vi "macro_DrumSeq_Continuous.vi"() -> ()   [LabVIEW 2019, in "Trajectory_Library.lvlib"]
uses:
  VI/BoolCmd_Recv_Internal.vi
  VI/DigSeqLogic_Edge_On.vi
  Util_GetTime.vi
  Timer_New.vi
  VI/BoolCmd_ObtainQueue.vi
  VI/Util_GetTime_U32.vi
  VI/Util_GetTime_U64.vi
  <vilib>/Utility/semaphor.llb/Obtain Semaphore Reference.vi
  Timer_Reset.vi
  VI/Timer_Restart.vi
  Timer_HasPeriodPassedOnce.vi
  Trajectory_Library.lvlib
panel:
  out "Some Speed demand":dbl
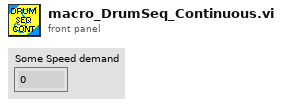
[diagram p1: front panel]
types:
  T1 = typedef "Trajectory_Library.lvlib/DrumSequence_Step_Enum.ctl" = enum16{"Do Nothing", "Step 1", "Step 2", "Step 3", "Step 4", "Step 5", "Step 6", "Step 7", "Step 8", "Step 9", "Step 10", "Step 11", "Step 12", "Step 13", "Step 14", "Step 15", "Step 16", "Step 17", "Step 18", "Step 19", "Step 20", "Step 21", "Step 22", "Step 23", "Step 24", "Step 25", "Step 26", "Step 27", "Step 28", "Step 29", "Step 30", "Step 31", "Step 32", "Cancel", "Initialize", "Error"}
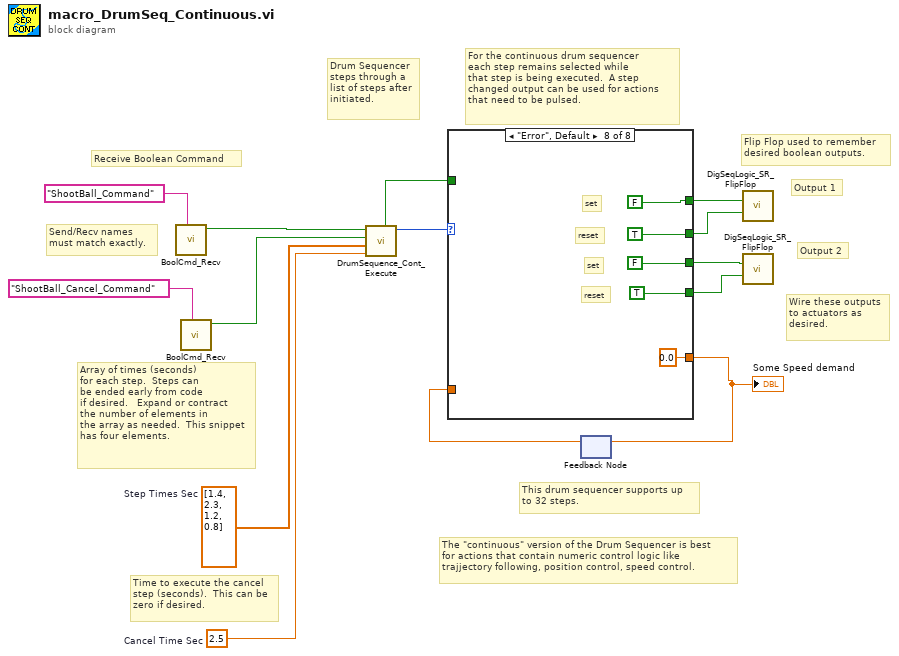
[diagram p0: block diagram]
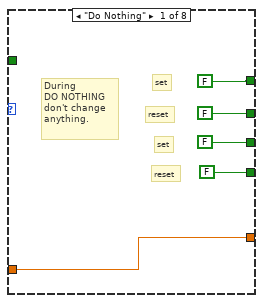
[diagram p2: hidden frame]
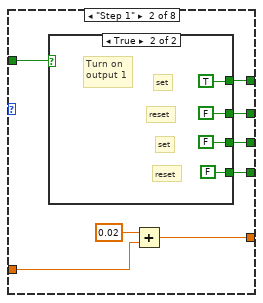
[diagram p3: hidden frame]
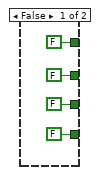
[diagram p4: hidden frame]
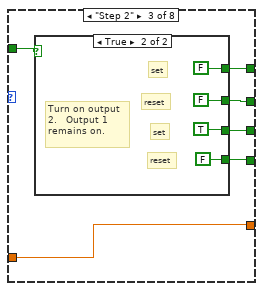
[diagram p5: hidden frame]
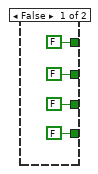
[diagram p6: hidden frame]
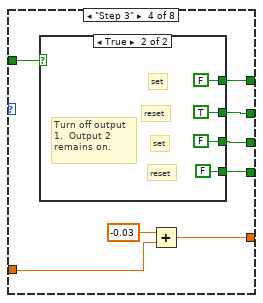
[diagram p7: hidden frame]
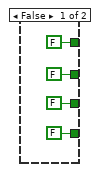
[diagram p8: hidden frame]
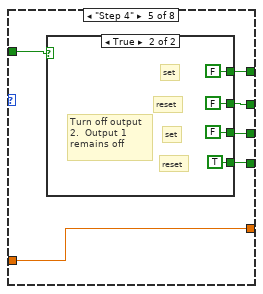
[diagram p9: hidden frame]
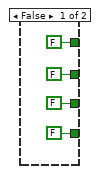
[diagram p10: hidden frame]
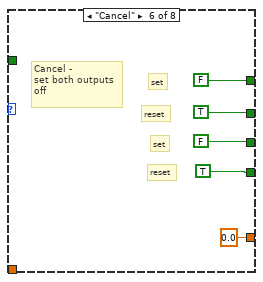
[diagram p11: hidden frame]
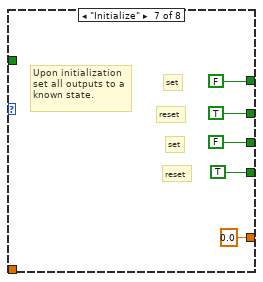
[diagram p12: hidden frame]
diagram:
  w9 = 2.5  # Cancel Time Sec
  w10 = dbl[] [1.4, 2.3, 1.2, 0.8]  # Step Times Sec
  # "This drum sequencer supports up\nto 32 steps."
  # "Wire these outputs\nto actuators as\ndesired."
  # "Output 2"
  # "Output 1"
  # "Flip Flop used to remember\ndesired boolean outputs."
  # "The \"continuous\" version of the Drum Sequencer is best\nfor actions that contain numeric control logic like \ntrajjectory following, position control, speed control."
  # "For the continuous drum sequencer\neach step remains selected while\nthat step is being executed.  A step\nchanged output can be used for actions\nthat need to be pulsed."
  # "Drum Sequencer\nsteps through a \nlist of steps after\ninitiated."
  # "Time to execute the cancel\nstep (seconds).  This can be\nzero if desired."
  # "Array of times (seconds)\nfor each step.  Steps can\nbe ended early from code\nif desired.   Expand or contract\nthe number of elements in\nthe array as needed.  This snippet\nhas four elements."
  # "Send/Recv names\nmust match exactly."
  # "Receive Boolean Command"
  n1 = call "BoolCmd_Recv.vi"("Command Name"="ShootBall_Command") -> ("New Request"=w13:bool)  [unwired: 9 in, 1 out]
  n2 = call "BoolCmd_Recv.vi"("Command Name"="ShootBall_Cancel_Command") -> ("New Request"=w11:bool)  [unwired: 9 in, 1 out]
  n3 = call "DrumSequence_Cont_Execute.vi"("Cancel Time Sec"=w9, "Step Times Sec"=w10, "Cancel"=w11, "Initiate"=w13) -> ("Step Number State"=w8:T1, "New Step"=w3:bool)  [unwired: 3 in, 3 out]
  n4 = feedback #1() -> (w1:dbl)  [unwired: 1 in]
  n5 = case shown="\"Error\", Default" w8 {
    tunnel: [FALSE w24 w38 w54 w68 FALSE FALSE FALSE] -> w7
    tunnel: [FALSE w25 w39 w55 w69 TRUE TRUE TRUE] -> w6
    tunnel: [FALSE w26 w40 w56 w70 FALSE FALSE FALSE] -> w5
    tunnel: [FALSE w27 w41 w57 w71 TRUE TRUE TRUE] -> w4
    tunnel: w3 -> [_ w23 w36 w50 w66 _ _ _]
    tunnel: [w15 w20 w37 w51 w67 0.0 0.0 0.0] -> w2
    tunnel: w1 -> [w15 w21 w37 w52 w67 _ _ _]
    frame "Do Nothing" {
      # "During \nDO NOTHING\ndon't change\nanything."
      # "reset"
      # "set"
      # "reset"
      # "set"
    }
    frame "Step 1" {
      n6 = case shown="True" w23 {
        tunnel: [FALSE FALSE] -> w27
        tunnel: [FALSE FALSE] -> w26
        tunnel: [FALSE FALSE] -> w25
        tunnel: [FALSE TRUE] -> w24
        frame False {
        }
        frame True {
          # "Turn on \noutput 1"
          # "reset"
          # "set"
          # "reset"
          # "set"
        }
      }
      n7 = Add(x=0.02, y=w21) -> (x+y=w20:dbl)
    }
    frame "Step 2" {
      n8 = case shown="True" w36 {
        tunnel: [FALSE FALSE] -> w41
        tunnel: [FALSE TRUE] -> w40
        tunnel: [FALSE FALSE] -> w39
        tunnel: [FALSE FALSE] -> w38
        frame False {
        }
        frame True {
          # "Turn on output\n2.   Output 1\nremains on."
          # "reset"
          # "set"
          # "reset"
          # "set"
        }
      }
    }
    frame "Step 3" {
      n9 = case shown="True" w50 {
        tunnel: [FALSE FALSE] -> w57
        tunnel: [FALSE FALSE] -> w56
        tunnel: [FALSE TRUE] -> w55
        tunnel: [FALSE FALSE] -> w54
        frame False {
        }
        frame True {
          # "Turn off output\n1.  Output 2\nremains on."
          # "reset"
          # "set"
          # "reset"
          # "set"
        }
      }
      n10 = Add(x=-0.03, y=w52) -> (x+y=w51:dbl)
    }
    frame "Step 4" {
      n11 = case shown="True" w66 {
        tunnel: [FALSE TRUE] -> w71
        tunnel: [FALSE FALSE] -> w70
        tunnel: [FALSE FALSE] -> w69
        tunnel: [FALSE FALSE] -> w68
        frame False {
        }
        frame True {
          # "Turn off output\n2.  Output 1\nremains off"
          # "reset"
          # "set"
          # "reset"
          # "set"
        }
      }
    }
    frame "Cancel" {
      # "Cancel - \nset both outputs\noff"
      # "reset"
      # "set"
      # "reset"
      # "set"
    }
    frame "Initialize" {
      # "reset"
      # "set"
      # "reset"
      # "set"
      # "Upon initialization\nset all outputs to a\nknown state."
    }
    frame "Error", Default {
      # "reset"
      # "set"
      # "reset"
      # "set"
    }
  }
  "Some Speed demand" <- w2
  n12 = feedback-in #1(w2) -> ()
  n13 = call "DigSeqLogic_SR_FlipFlop.vi"("Set"=w7, "Reset"=w6) -> ()  [unwired: 12 in, 2 out]
  n14 = call "DigSeqLogic_SR_FlipFlop.vi"("Set"=w5, "Reset"=w4) -> ()  [unwired: 12 in, 2 out]
